vi "setPinnedRobots.vi"(8 "error in (no error)":errorcluster, 9 "Defensive ids":dbl[](array[numeric]), 10 "Offensive ids":dbl[](array[numeric]), 11 "Game in":refnum<class "Game.lvclass">) -> (0 "error out":errorcluster, 3 "Game out":refnum<class "Game.lvclass">)   [LabVIEW 2023, in "Game.lvclass"]
uses:
  Game.lvclass
  Game.lvclass/Game.ctl
  Write Offensive ids.vi
  Write Defensive ids.vi
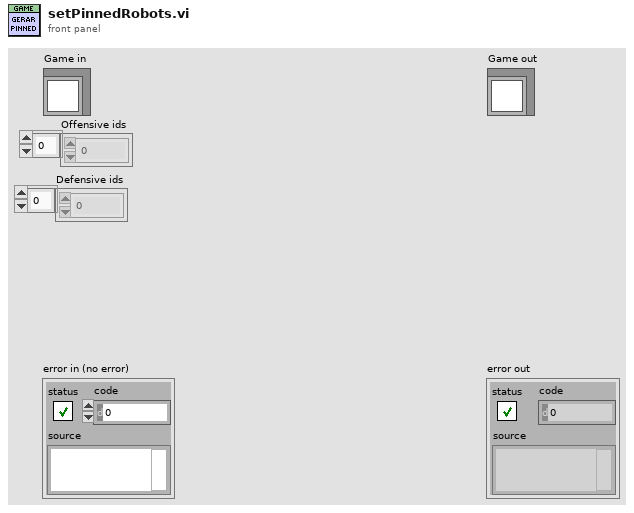
[diagram p1: front panel]
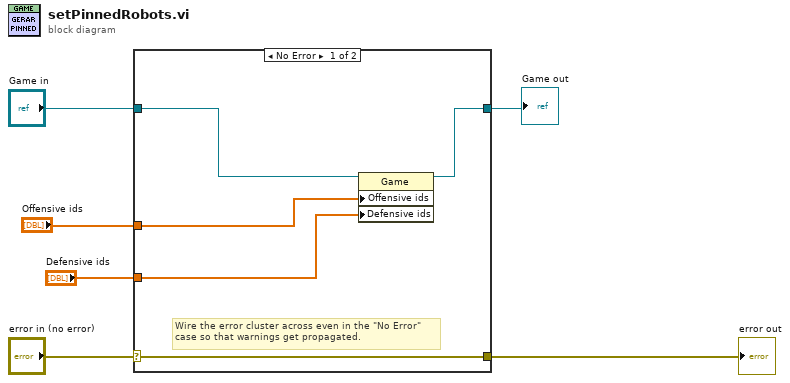
[diagram p0: block diagram]
diagram:
  n1 = case shown="No Error" "error in (no error)" {
    selector: "error in (no error)" -> [w11 w13]
    tunnel: [w11 w13] -> w5
    tunnel: [w10 w12] -> w3
    tunnel: "Game in" -> [w9 w12]
    tunnel: "Offensive ids" -> [w8 _]
    tunnel: "Defensive ids" -> [w7 _]
    frame No Error {
      # "Wire the error cluster across even in the \"No Error\"\ncase so that warnings get propagated."
      n2 = property class="Game"(reference=w9, "Offensive ids"=w8, "Defensive ids"=w7) -> (reference out=w10:refnum<class "Game.lvclass">)  [unwired: 1 in, 1 out]
    }
    frame Error {
    }
  }
  "error out" <- w5
  "Game out" <- w3
